vi "receiveTemperatureData.vi"(8 "error in (no error)":errorcluster, 11 "Model in":refnum<class "Model.lvclass">) -> (0 "error out":errorcluster, 3 "Model out":refnum<class "Model.lvclass">)   [LabVIEW 2013, in "Model.lvclass"]
uses:
  Model.lvclass
  Model.lvclass/Model.ctl
  ApplicationElements/Log/TestDataLog/TestDataLog.lvclass/TestDataLog.ctl
  <userlib>/Common/Devices/FlukeDMM/FlukeDMM/FlukeDMM.lvclass/FlukeDMM.ctl
  ApplicationElements/Log/TestDataLog/TestDataLog.lvclass
  <userlib>/Common/Devices/FlukeDMM/FlukeDMM/FlukeDMM.lvclass
  ApplicationElements/TestMonitor/TestMonitor.lvclass
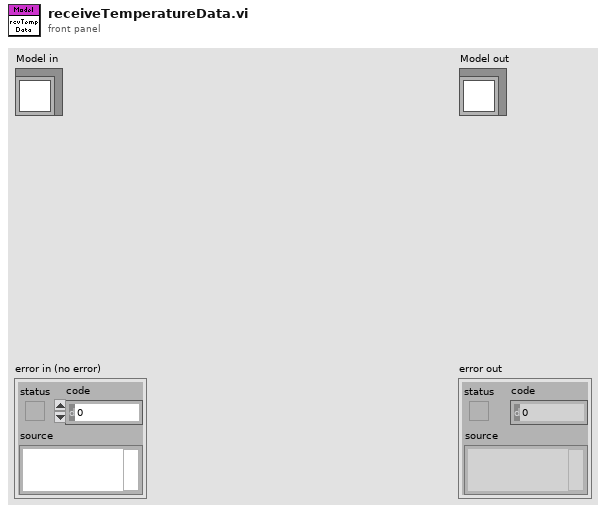
[diagram p1: front panel]
types:
  T1 = typedef "AITDTTypedefs.lvlib/InputData.ctl" = cluster{"Temperature Measured":dbl[unit], "ADCs":T2}
  T2 = typedef "ILCCommon.lvlib/ILCTypedefs.lvlib/ADCs.ctl" = cluster{"Ch0":i32, "Ch1":i32, "Ch2":i32, "Ch3":i32, "Ch4":i32}
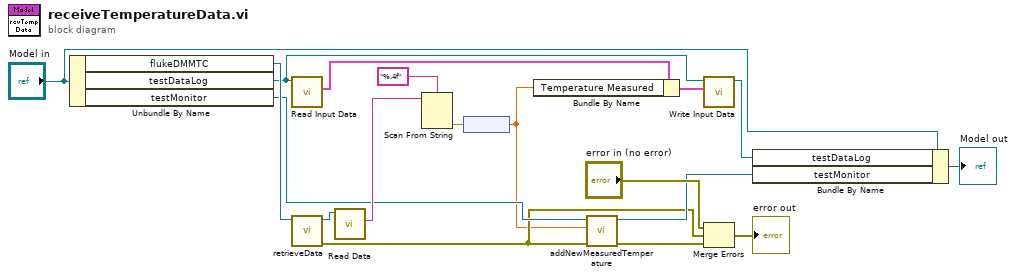
[diagram p0: block diagram]
diagram:
  n1 = Unbundle By Name("Model in") -> ("flukeDMMTC"=w12:refnum<class "FlukeDMMTC.lvclass">, "testDataLog"=w2:refnum<class "TestDataLog.lvclass">, "testMonitor"=w7:refnum<class "TestMonitor.lvclass">)
  n2 = call "Read Input Data.vi"("TestDataLog in"=w2) -> ("Input Data"=w1:T1)  [unwired: 9 in, 1 out]
  n3 = call <userlib>:"retrieveData.vi"("FlukeDMM in"=w12) -> ("error out"=w5:errorcluster, "FlukeDMM out"=w11:refnum<class "FlukeDMMTC.lvclass">)  [unwired: 9 in]
  n4 = call <userlib>:"Read Data.vi"("FlukeDMM in"=w11) -> ("Data"=w10:string)  [unwired: 9 in, 1 out]
  n5 = Scan From String(format string="%.4f", input string=w10) -> (output 1=w8:dbl)  [unwired: 3 in, 3 out]
  n6 = node(w8) -> (w3:dbl[unit])
  n7 = Bundle By Name(cluster=w1, "Temperature Measured"=w3) -> (w13:T1)
  n8 = call "addNewMeasuredTemperature.vi"("error in (no error)"=w5, "Temperature Measured"=w3, "TestMonitor in"=w7) -> ("error out"=w4:errorcluster, "TestMonitor out"=w6:refnum<class "TestMonitor.lvclass">)  [unwired: 7 in]
  n9 = call "Write Input Data.vi"("Input Data"=w13, "Logger in"=w2) -> ("Logger out"=w14:refnum<class "TestDataLog.lvclass">)  [unwired: 9 in]
  n10 = Merge Errors("error in (no error)", w5, w4) -> (→"error out":errorcluster)
  n11 = Bundle By Name(cluster="Model in", "testDataLog"=w14, "testMonitor"=w6) -> (→"Model out":refnum<class "Model.lvclass">)
